vi "Get Terminals Info.vi"(8 "error in (no error)":errorcluster, 10 "structure name":string, 11 "Terms[]":refnum<vi>[](array[refnum])) -> (0 "error out":errorcluster, 3 "output cluster":T1)   [LabVIEW 2014]
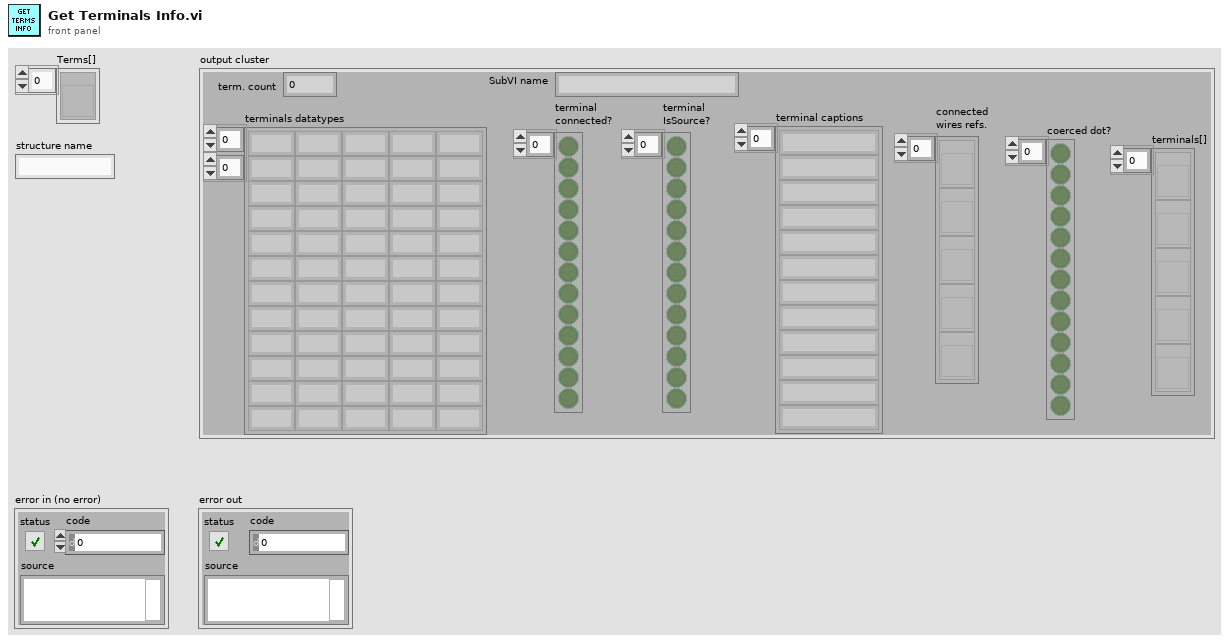
[diagram p1: front panel]
types:
  T1 = cluster{"terminals datatypes":string[][], "terminal\nconnected?":bool[], "terminal captions":string[], "term. count":i32, "terminal\nIsSource?":bool[], "SubVI name":string, "connected\nwires refs.":refnum<vi>[], "coerced dot?":bool[], "terminals[]":refnum<vi>[]}
  T2 = cluster{"terminals datatypes":string[][], "terminal connected?":bool[], "terminal captions":string[], "term. count":i32, "terminal IsSource":bool[], "structure name":string, "connected wires refs.":refnum<vi>[], "coercetd dot?":bool[], "terminals[]":refnum<vi>[]}
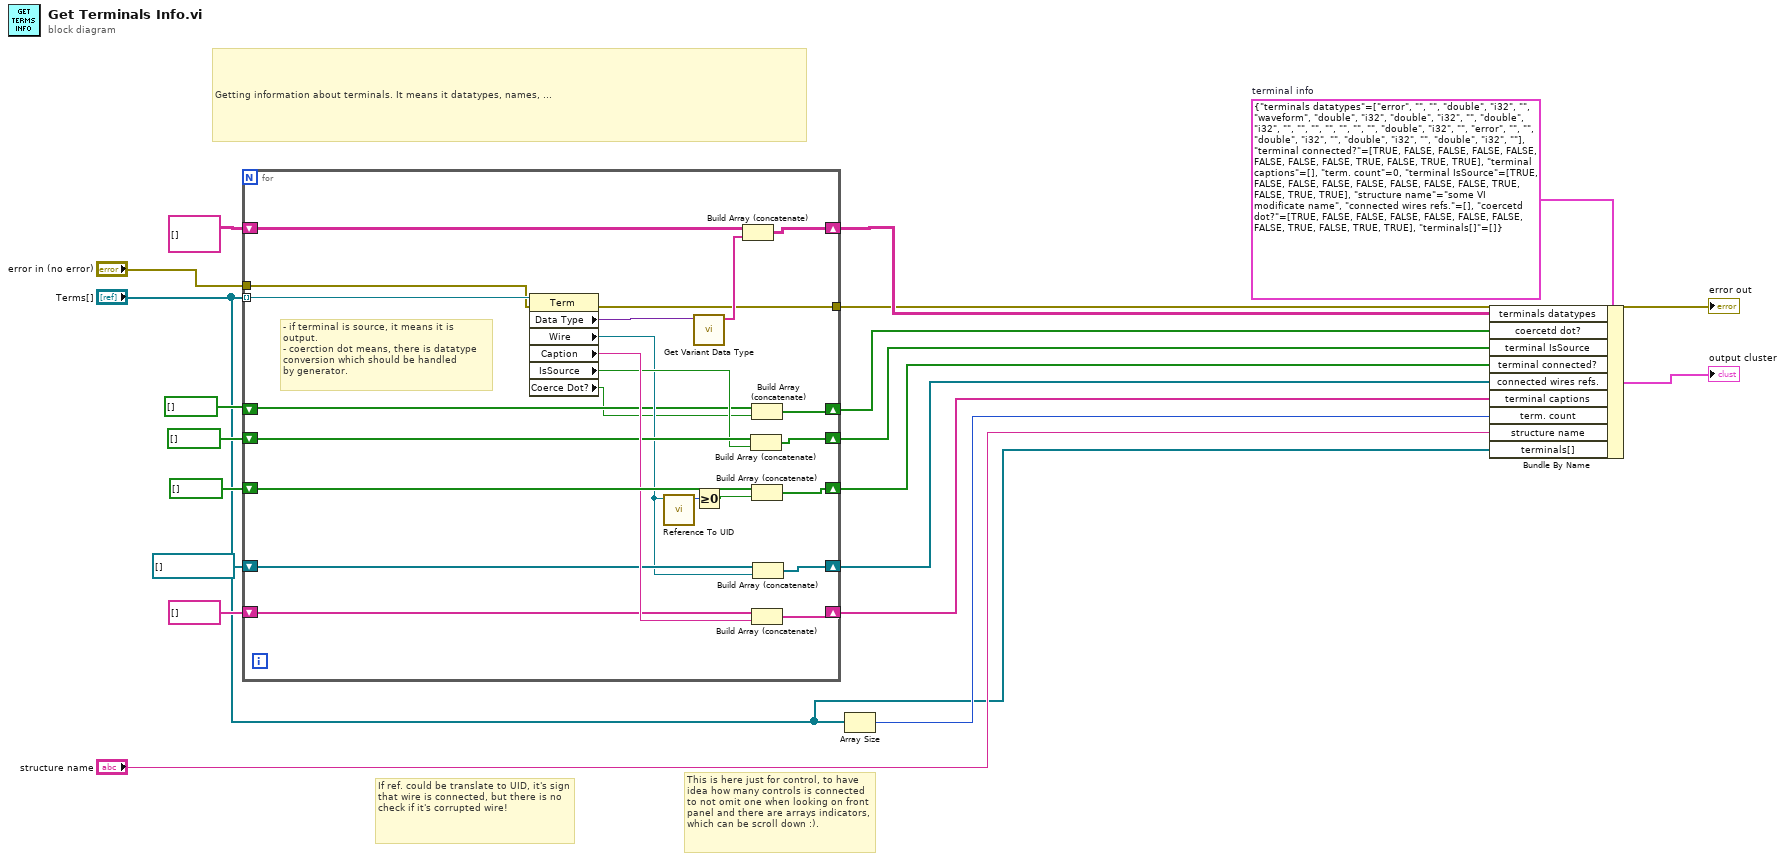
[diagram p0: block diagram]
diagram:
  w9 = T2 {"terminals datatypes"=[["error", "", ""], ["double", "i32", ""], ["waveform", "double", "i32"], ["double", "i32", ""], ["double", "i32", ""], ["", "", ""], ["", "", ""], ["double", "i32", ""], ["error", "", ""], ["double", "i32", ""], ["double", "i32", ""], ["double", "i32", ""]], "terminal connected?"=[TRUE, FALSE, FALSE, FALSE, FALSE, FALSE, FALSE, FALSE, TRUE, FALSE, TRUE, TRUE], "terminal captions"=[], "term. count"=0, "terminal IsSource"=[TRUE, FALSE, FALSE, FALSE, FALSE, FALSE, FALSE, FALSE, TRUE, FALSE, TRUE, TRUE], "structure name"="some VI modificate name", "connected wires refs."=[], "coercetd dot?"=[TRUE, FALSE, FALSE, FALSE, FALSE, FALSE, FALSE, FALSE, TRUE, FALSE, TRUE, TRUE], "terminals[]"=[]}  # terminal info
  # "If ref. could be translate to UID, it's sign that wire is connected, but there is no check if it's corrupted wire!"
  # "This is here just for control, to have idea how many controls is connected to not omit one when looking on front panel and there are arrays indicators, which can be scroll down :)."
  # "Getting information about terminals. It means it datatypes, names, ..."
  n1 = for {
    tunnel: "Terms[]" -> [w40] mode=indexing
    shift-right: [w41] -> w6
    shift-left: string[][] [] -> [w42]
    tunnel: "error in (no error)" -> [w37]
    tunnel: [w36] -> w4
    shift-right: [w34] -> w7
    shift-left: bool[] [] -> [w35]
    shift-right: [w31] -> w8
    shift-left: string[] [] -> [w30]
    shift-right: [w23] -> w11
    shift-left: bool[] [] -> [w29]
    shift-right: [w26] -> w16
    shift-left: refnum<vi>[] [] -> [w25]
    shift-right: [w22] -> w18
    shift-left: bool[] [] -> [w21]
    # "- if terminal is source, it means it is output.\n- coerction dot means, there is datatype\nconversion which should be handled\nby generator."
    n2 = property class="Term"(reference=w40, error in=w37) -> (error out=w36:errorcluster, "Data Type"=w39:variant, "Wire"=w24:refnum<vi>, "Caption"=w32:string, "IsSource"=w28:bool, "Coerce Dot?"=w20:bool)  [unwired: 1 out]
    n3 = call "Reference To UID.vi"("Reference"=w24) -> ("UID"=w33:i32)  [unwired: 10 in]
    n4 = call "Get Variant Data Type.vi"("Variant in"=w39) -> ("Data Types[]"=w38:string[])  [unwired: 9 in, 1 out]
    n5 = Greater Or Equal To 0?(x=w33) -> (x >= 0?=w27:bool)
    n6 = Build Array (concatenate)(w42, w38) -> (w41:string[][])
    n7 = Build Array (concatenate)(w29, w28) -> (w23:bool[])
    n8 = Build Array (concatenate)(w21, w20) -> (w22:bool[])
    n9 = Build Array (concatenate)(w35, w27) -> (w34:bool[])
    n10 = Build Array (concatenate)(w30, w32) -> (w31:string[])
    n11 = Build Array (concatenate)(w25, w24) -> (w26:refnum<vi>[])
  }
  "error out" <- w4
  n12 = Array Size(array="Terms[]") -> (size(s)=w15:i32)
  n13 = Bundle By Name(cluster=w9, "terminals datatypes"=w6, "coercetd dot?"=w18, "terminal IsSource"=w11, "terminal connected?"=w7, "connected wires refs."=w16, "terminal captions"=w8, "term. count"=w15, "structure name"="structure name", "terminals[]"="Terms[]") -> (→"output cluster":T2)
